vi "Close.vi"(8 "error in":errorcluster, 11 "CANopen Master in":refnum<class "CANopen Master.lvclass">) -> (0 "error out":errorcluster, 3 "CANopen Master out":refnum<class "CANopen Master.lvclass">)   [LabVIEW 2024, in "CANopen Master.lvlib" / "CANopen Master.lvclass"]
uses:
  CANopen Master.lvclass
  CANopen Master.lvclass/CANopen Master.ctl
  Network Mangement/Network Mangement.lvclass
  SDO Manager/SDO Manager.lvclass
  Heartbeat/Heartbeat.lvclass
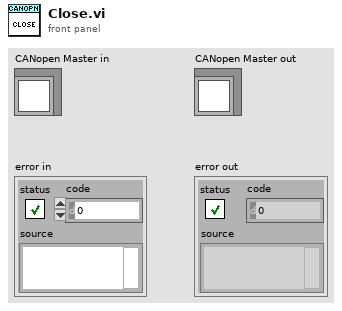
[diagram p1: front panel]
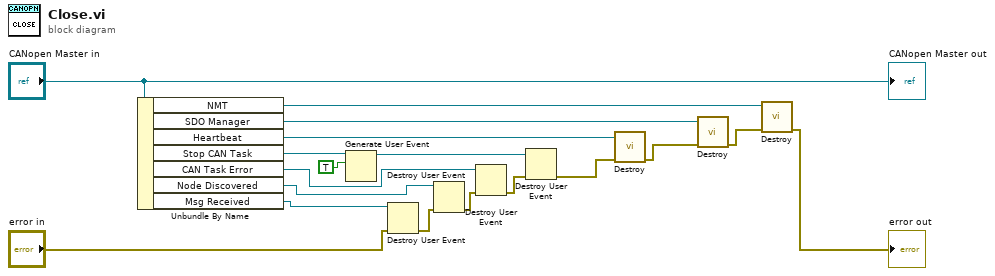
[diagram p0: block diagram]
diagram:
  n1 = Unbundle By Name("CANopen Master in") -> ("NMT"=w14:refnum<class "Network Mangement.lvclass">, "SDO Manager"=w16:refnum<class "SDO Manager.lvclass">, "Heartbeat"=w17:refnum<class "Heartbeat.lvclass">, "Stop CAN Task"=w7:refnum<user-event>, "CAN Task Error"=w5:refnum<user-event>, "Node Discovered"=w4:refnum<user-event>, "Msg Received"=w1:refnum<user-event>)
  n2 = Generate User Event(user event=w7, event data cluster=TRUE ("event data")) -> (user event out=w6:refnum<user-event>)  [unwired: 2 in, 1 out]
  n3 = Destroy User Event(user event=w1, error in="error in") -> (error out=w8:errorcluster)
  n4 = Destroy User Event(user event=w4, error in=w8) -> (error out=w2:errorcluster)
  n5 = Destroy User Event(user event=w5, error in=w2) -> (error out=w11:errorcluster)
  n6 = Destroy User Event(user event=w6, error in=w11) -> (error out=w10:errorcluster)
  n7 = call-dynamic "Destroy.vi"("Error In"=w10, "reference in"=w17) -> ("Error Out"=w15:errorcluster)  [unwired: 8 in, 1 out]
  n8 = call-dynamic "Destroy.vi"("Error In"=w15, "reference in"=w16) -> ("Error Out"=w13:errorcluster)  [unwired: 8 in, 1 out]
  n9 = call-dynamic "Destroy.vi"("Error In"=w13, "reference in"=w14) -> ("Error Out"=→"error out":errorcluster)  [unwired: 8 in, 1 out]
  "CANopen Master out" <- "CANopen Master in"
